vi "Program_Ini.vi"() -> ()   [LabVIEW 2019]
uses:
  <vilib>/addons/control/pid/pid.llb/PID (DBL).vi
  <vilib>/addons/control/pid/NI_PID_pid.lvlib
panel:
  out "expo":string
  out "den":string
  out "num":string
  in  "Retardo":dbl
  out "Grafica":cluster{"Y":dbl, "U":dbl}(graph)
  in  "Lazo cerrado":bool
  in  "Set point":dbl
  out "n":i32
  out "Y":dbl format="%.2f"
  in  "Entrada\nescalon":dbl
  in  "Dt":dbl
  in  "Den":dbl[](array[numeric])
  in  "Num":dbl[](array[numeric])
  # "Lazo abierto"
  # "Y(S)"
  # "="
  # "U(S)"
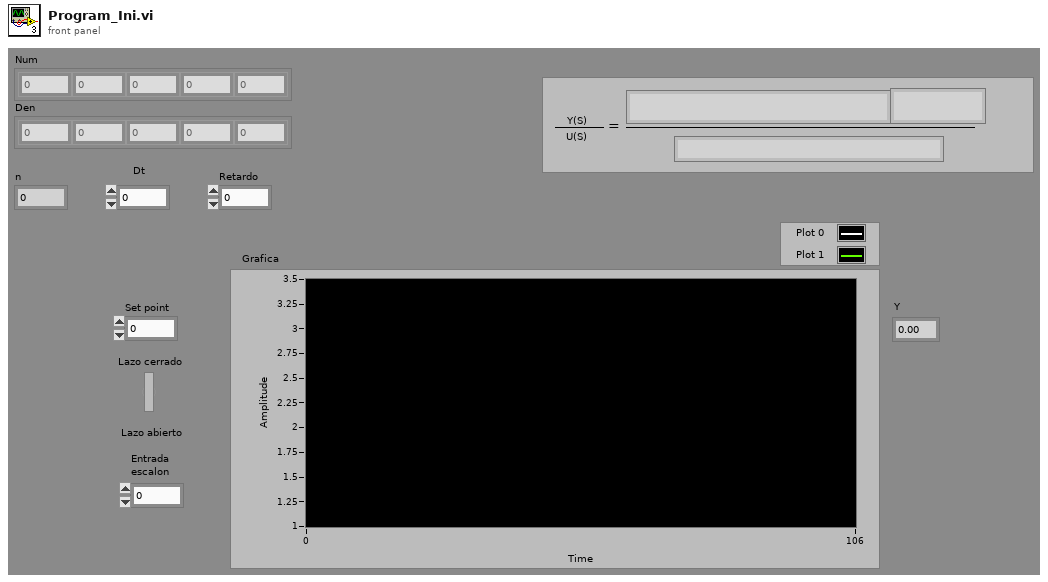
[diagram p1: front panel]
types:
  T1 = cluster{"proportional gain (Kc)":dbl, "integral time (Ti, min)":dbl, "derivative time (Td, min)":dbl}
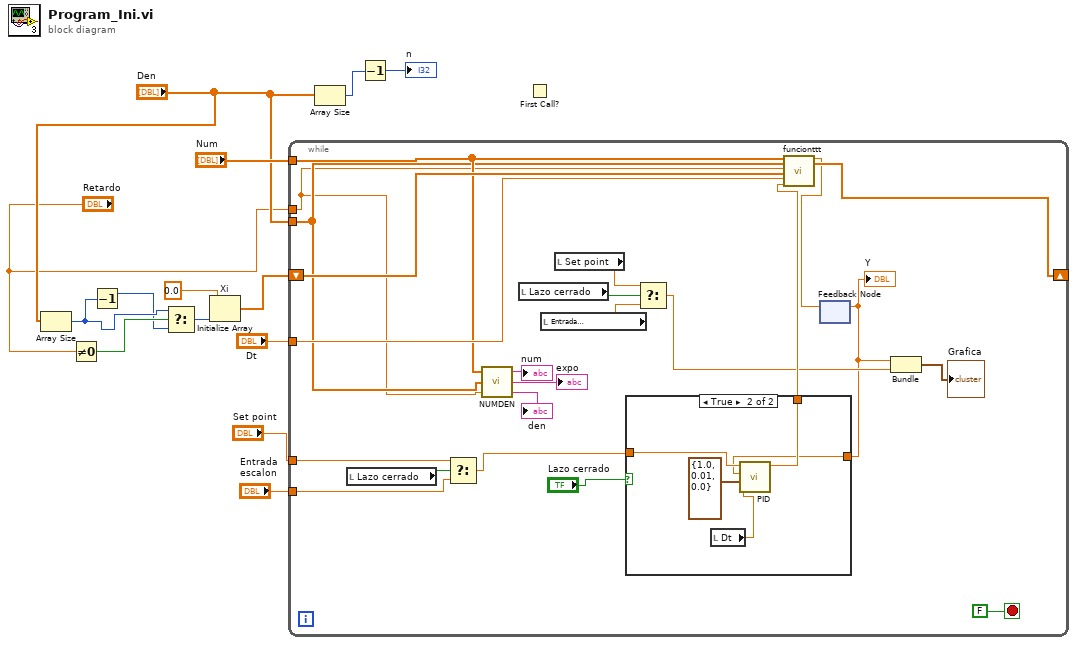
[diagram p0: block diagram]
diagram:
  n1 = Array Size(array="Den") -> (size(s)=w4:i32)
  n2 = Not Equal To 0?(x="Retardo") -> (x != 0?=w3:bool)
  n3 = Decrement(x=w4) -> (x-1=w1:i32)
  n4 = Select(t=w4, s=w3, f=w1) -> (s? t:f=w2:i32)
  n5 = Initialize Array "Xi"(0.0 ("element"), w2) -> (w12:dbl[])
  n6 = while {
    tunnel: "Num" -> [w18]
    tunnel: "Den" -> [w17]
    shift-right: [w30] -> _
    shift-left: w12 -> [w37]
    tunnel: "Dt" -> [w21]
    tunnel: "Set point" -> [w35]
    tunnel: "Entrada\nescalon" -> [w34]
    tunnel: "Retardo" -> [w16]
    stop <- FALSE stop-if-true
    n7 = local read "Lazo cerrado"() -> (w32:bool)
    n8 = Select(t=w35, s=w32, f=w34) -> (s? t:f=w29:dbl)
    n9 = call "NUMDEN.vi"("Retardo"=w16, "DENOMINADOR"=w17, "NUMERADOR"=w18) -> ("den"=→"den":string, "expo"=→"expo":string, "num"=→"num":string)
    n10 = local read "Lazo cerrado"() -> (w25:bool)
    n11 = local read "Entrada\nescalon"() -> (w27:dbl)
    n12 = local read "Set point"() -> (w26:dbl)
    n13 = Select(t=w26, s=w25, f=w27) -> (s? t:f=w24:dbl)
    n14 = feedback #1() -> (w23:dbl)  [unwired: 1 in]
    "Y" <- w23
    n15 = case shown="True" "Lazo cerrado" {
      tunnel: w29 -> [w38 w41]
      tunnel: [w38 w40] -> w31
      tunnel: w23 -> [_ w39]
      frame False {
      }
      frame True {
        n16 = local read "Dt"() -> (w43:dbl)
        n17 = call-poly <vilib>:"PID.vi"("dt (s)"=w43, "PID gains"=T1 {"proportional gain (Kc)"=1.0, "integral time (Ti, min)"=0.01, "derivative time (Td, min)"=0.0}, "process variable"=w39, "setpoint"=w41) -> ("output"=w40:dbl)  [unwired: 6 in, 1 out]
      }
    }
    n18 = call "funcionttt.vi"("Num"=w18, "Den"=w17, "Retardo"=w16, "XINIT"=w37, "DT"=w21, "U"=w31) -> ("Y"=w28:dbl, "Out"=w30:dbl[])  [unwired: 12 in]
    n19 = feedback-in #1(w28) -> ()
    n20 = Bundle("Y"=w23, "Entrada\nescalon"=w24) -> (→"Grafica":cluster{"Y":dbl, "Entrada\nescalon":dbl})  [unwired: 1 in]
  }
  n21 = Array Size(array="Den") -> (size(s)=w10:i32)
  n22 = Decrement(x=w10) -> (x-1=→"n":i32)
  n23 = First Call?() -> ()  [unwired: 1 out]
